vi "Browse.vi"(7 "Current Strings and Values":T1, 8 "error in (no error)":errorcluster, 10 "Current Value":string, 11 "Dynamic Values in":refnum<class "Dynamic Values.lvclass">) -> (0 "error out":errorcluster, 1 "Cancelled?":bool, 2 "Selected Value":string, 3 "Dynamic Values out":refnum<class "Dynamic Values.lvclass">, 5 "Strings and Values []":T1)   [LabVIEW 2020, in "Dynamic Combobox.lvlib" / "Dynamic Values.lvclass"]
uses:
  Dynamic Values.lvclass
  <vilib>/Utility/miscctls.llb/LVComboBoxStrsAndValuesArrayTypeDef.ctl
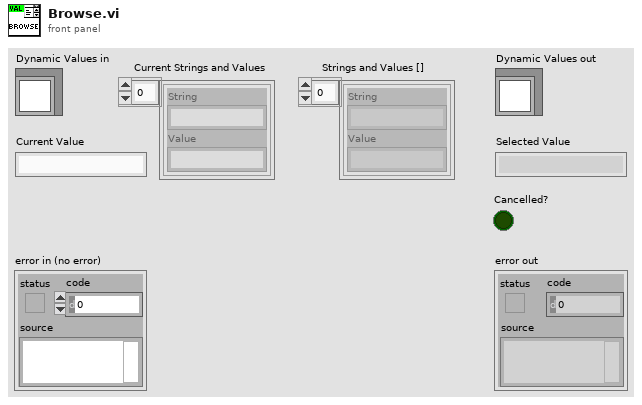
[diagram p1: front panel]
types:
  T1 = typedef "LVComboBoxStrsAndValuesArrayTypeDef.ctl" = cluster{"String":string, "Value":string}[]
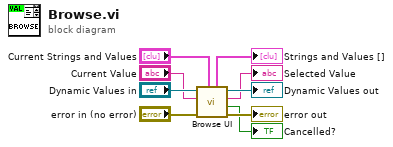
[diagram p0: block diagram]
diagram:
  n1 = call "Browse UI.vi"("Current Strings and Values"="Current Strings and Values", "error in (no error)"="error in (no error)", "Current Value"="Current Value", "Dynamic Values in"="Dynamic Values in") -> ("error out"=→"error out":errorcluster, "Cancelled?"=→"Cancelled?":bool, "Selected Value"=→"Selected Value":string, "Dynamic Values out"=→"Dynamic Values out":refnum<class "Dynamic Values.lvclass">, "Strings and Values []"=→"Strings and Values []":T1)  [unwired: 3 in]
